vi "event queue parser.vi"(11 "Status":T1 {"Setting"."X Pos." scale=-2.0..2.0; "Setting"."Y Pos." scale=-2.0..2.0}) -> (1 "Data":string, 2 "Event":T4, 3 "队列输出":refnum<queue>)   [LabVIEW 2013]
uses:
  event-package.ctl
  Event1.ctl
  init-status.ctl
  Setting.ctl
  data-package.ctl
  Event.ctl
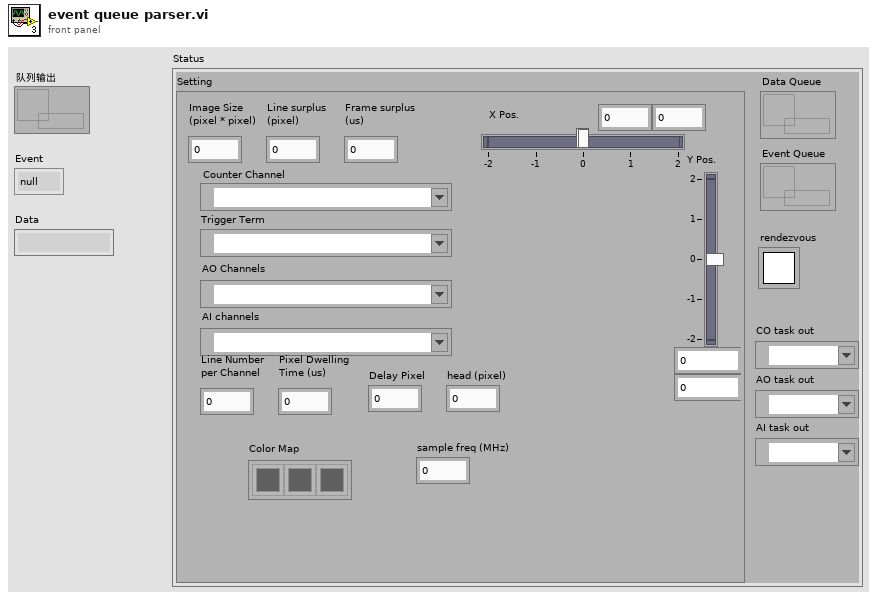
[diagram p1: front panel]
types:
  T1 = typedef "init-status.ctl" = cluster{"Setting":T2, "Event Queue":refnum<queue>, "Data Queue":refnum<queue>, "rendezvous":T3, "CO task out":refnum<k21>, "AO task out":refnum<k21>, "AI task out":refnum<k21>}
  T2 = typedef "Setting.ctl" = cluster{"Image Size\n(pixel * pixel)":i32, "Counter Channel":tag, "Trigger Term":tag, "AO Channels":tag, "Y Pos.":cluster{dbl, dbl}, "X Pos.":cluster{dbl, dbl}, "Line surplus\n(pixel)":i32, "Frame surplus\n(us)":i32, "AI channels":tag, "Line Number\nper Channel":i32, "Delay Pixel":i32, "Pixel Dwelling\nTime (us)":i32, "Color Map":u32[], "head (pixel)":i32, "sample freq (MHz)":dbl}
  T3 = typedef "Rendezvous RefNum" = refnum<k1>
  T4 = typedef "Event1.ctl" = enum16{"null", "stop AI", "stop AO", "stop Imaging", "stop Counter", "save sheet", "restart", "save tiff", "gain/offset changed", "save multiple tiffs"}
  T5 = typedef "event-package.ctl" = cluster{"Event":T4, "Data":string}
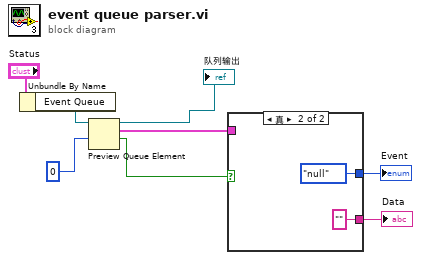
[diagram p0: block diagram]
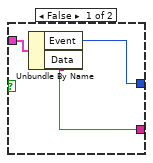
[diagram p2: hidden frame]
diagram:
  n1 = Unbundle By Name("Status") -> ("Event Queue"=w1:refnum<queue>)
  n2 = Preview Queue Element(queue=w1, timeout in ms (-1)=0 ("超时毫秒(-1)")) -> (queue out=→"队列输出":refnum<queue>, element=w5:T5, timed out?=w3:bool)  [unwired: 1 in, 1 out]
  n3 = case shown="真" w3 {
    tunnel: [w11 "" ("Data")] -> w8
    tunnel: [w10 Event1."null" ("Event")] -> w6
    tunnel: w5 -> [w9 _]
    frame False {
      n4 = Unbundle By Name(w9) -> ("Event"=w10:T4, "Data"=w11:string)
    }
    frame True {
    }
  }
  "Data" <- w8
  "Event" <- w6
